vi "Connect Channels (Multiple).vi"(8 "error in (no error)":errorcluster, 10 "connection list":string, 11 "SLSC Switch in":refnum<class "SLSC Switch.lvclass">) -> (0 "error out":errorcluster, 3 "SLSC Switch out":refnum<class "SLSC Switch.lvclass">)   [LabVIEW 2015, in "SLSC Switch.lvclass"]
uses:
  SLSC Switch.lvclass
  Route Manager/Route Manager.lvclass
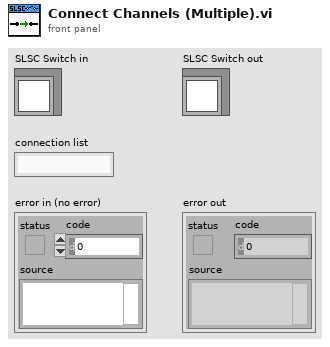
[diagram p1: front panel]
types:
  T1 = typedef "Route Manager.lvclass/Connection.ctl" = cluster{"channel 1":string, "channel 2":string}
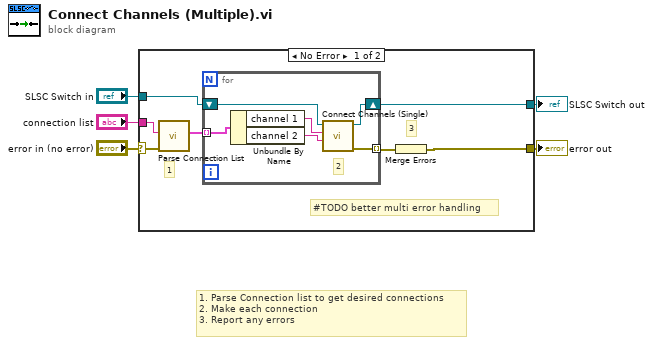
[diagram p0: block diagram]
diagram:
  # "1. Parse Connection list to get desired connections\n2. Make each connection\n3. Report any errors"
  n1 = case shown="No Error" "error in (no error)" {
    selector: "error in (no error)" -> [w8 w20]
    tunnel: [w7 w20] -> w4
    tunnel: [w12 w19] -> w2
    tunnel: "SLSC Switch in" -> [w11 w19]
    tunnel: "connection list" -> [w10 _]
    frame No Error {
      # "#TODO better multi error handling"
      # "3"
      # "1"
      n2 = call "Parse Connection List.vi"("error in (no error)"=w8, "connection list"=w10) -> ("connections"=w9:T1[])  [unwired: 8 in, 1 out]
      n3 = for {
        shift-right: [w18] -> w12
        shift-left: w11 -> [w17]
        tunnel: w9 -> [w16] mode=indexing
        tunnel: [w13] -> w6 mode=indexing
        # "2"
        n4 = Unbundle By Name(w16) -> ("channel 1"=w15:string, "channel 2"=w14:string)
        n5 = call "Connect Channels (Single).vi"("channel 2"=w14, "channel 1"=w15, "SLSC Switch in"=w17) -> ("error out"=w13:errorcluster, "SLSC Switch out"=w18:refnum<class "SLSC Switch.lvclass">)  [unwired: 7 in]
      }
      n6 = Merge Errors(w6) -> (w7:errorcluster)
    }
    frame Error {
    }
  }
  "error out" <- w4
  "SLSC Switch out" <- w2
